vi "Module Type.vi"(11 "Remote Messaging Module in":refnum<class "Remote Messaging Module.lvclass">) -> (2 "Module Type":string)   [LabVIEW 2020, in "Volatus.lvlib" / "Remote Messaging Module.lvclass"]
uses:
  Remote Messaging Module.lvclass
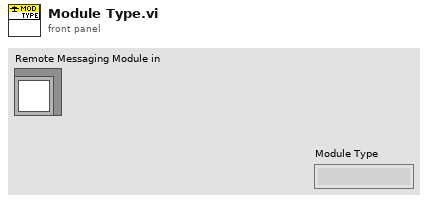
[diagram p1: front panel]
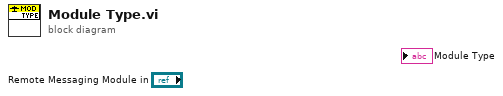
[diagram p0: block diagram]
diagram:
